vi "Configure DAQ.vi"(8 "error in (no error)":errorcluster, 11 "DAQ Module ID":i32) -> (0 "error out":errorcluster)   [LabVIEW 2020]
doc: "Configures inputs/outputs of the DAQ device. Naming and function of the ports is included in the VI."
uses:
  NI_DAQ/Libraries/NI DAQ/Controls/AI config parameters--cluster.ctl
  NI_DAQ/Libraries/NI DAQ/Controls/CI config parameters--cluster.ctl
  NI_DAQ/Libraries/NI DAQ/NI DAQ.lvlib
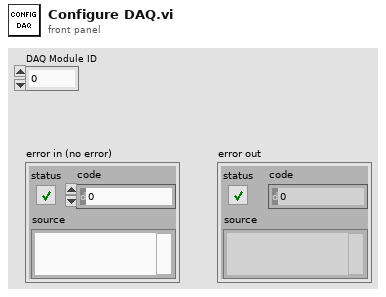
[diagram p1: front panel]
types:
  T1 = typedef "NI DAQ.lvlib/CI config parameters--cluster.ctl" = cluster{"Initial count":u32, "Count direction":i32, "Edge":i32}
  T2 = typedef "NI DAQ.lvlib/AI config parameters--cluster.ctl" = cluster{"Terminal configuration":i32, "min value":dbl, "max value":dbl}
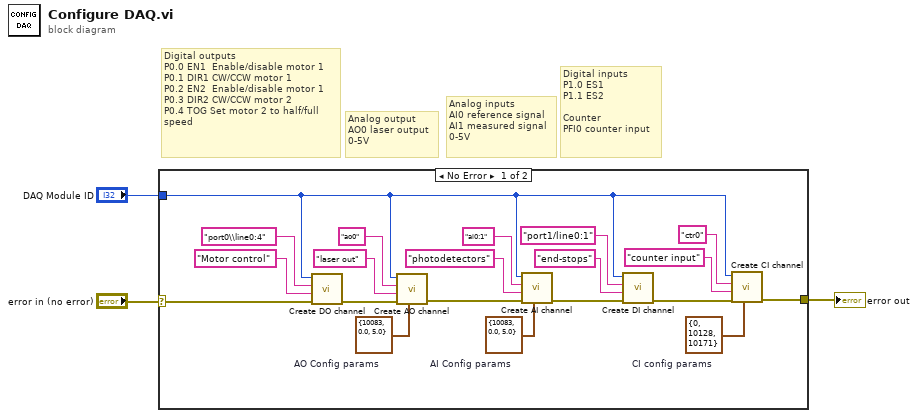
[diagram p0: block diagram]
diagram:
  # "Digital inputs\nP1.0 ES1\nP1.1 ES2\n\nCounter\nPFI0 counter input"
  # "Analog inputs\nAI0 reference signal\nAI1 measured signal\n0-5V"
  # "Analog output\nAO0 laser output\n0-5V"
  # "Digital outputs\nP0.0 EN1  Enable/disable motor 1\nP0.1 DIR1 CW/CCW motor 1\nP0.2 EN2  Enable/disable motor 1\nP0.3 DIR2 CW/CCW motor 2 \nP0.4 TOG Set motor 2 to half/full speed"
  n1 = case shown="No Error" "error in (no error)" {
    selector: "error in (no error)" -> [w12 w24]
    tunnel: [w10 w24] -> w2
    tunnel: "DAQ Module ID" -> [w9 _]
    frame No Error {
      w4 = T1 {"Initial count"=0, "Count direction"=10128, "Edge"=10171}  # CI config params
      w5 = T2 {"Terminal configuration"=10083, "min value"=0.0, "max value"=5.0}  # AI Config params
      w6 = T2 {"Terminal configuration"=10083, "min value"=0.0, "max value"=5.0}  # AO Config params
      n2 = call "Create DO channel.vi"("error in"=w12, "Channel name"="Motor control", "lines"="port0\\line0:4" ("Channel name"), "Module ID"=w9) -> ("error out"=w15:errorcluster)  [unwired: 7 in]
      n3 = call "Create AO channel.vi"("Config params"=w6, "error in"=w15, "Channel name"="laser out", "Physical channel"="ao0", "Module ID"=w9) -> ("error out"=w18:errorcluster)  [unwired: 6 in]
      n4 = call "Create AI channel.vi"("Config params"=w5, "error in"=w18, "Channel name"="photodetectors", "Physical channel"="ai0:1", "Module ID"=w9) -> ("error out"=w21:errorcluster)  [unwired: 6 in]
      n5 = call "Create DI channel.vi"("error in"=w21, "Channel name"="end-stops", "Physical channel"="port1/line0:1", "Module ID"=w9) -> ("error out"=w11:errorcluster)  [unwired: 7 in]
      n6 = call "Create CI channel.vi"("Channel config 2"=w4, "error in"=w11, "Channel name"="counter input", "Physical channel"="ctr0", "Module ID"=w9) -> ("error out"=w10:errorcluster)  [unwired: 6 in]
    }
    frame Error {
    }
  }
  "error out" <- w2
